vi "Initialise Standard Display.vi"() -> (3 "Standard Display Configuration out":refnum<class "Standard Display Configuration.lvclass">)   [LabVIEW 2016, in "Assert API Components.lvlib" / "Assert Display.lvlib" / "Main Display.lvlib" / "Standard Display Configuration.lvclass"]
uses:
  Standard Display Configuration.lvclass
  Standard Display Configuration.lvclass/Standard Display Configuration.ctl
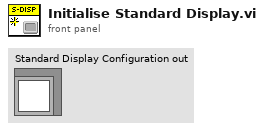
[diagram p1: front panel]
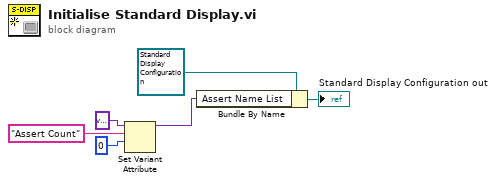
[diagram p0: block diagram]
diagram:
  n1 = Set Variant Attribute(Variant=variant ("Assert Name List"), name="Assert Count", value=0) -> (Variant out=w3:variant)  [unwired: 1 in, 2 out]
  n2 = Bundle By Name(cluster=refnum<class "Standard Display Configuration.lvclass"> refnum ("Standard Display Configuration in"), "Assert Name List"=w3) -> (→"Standard Display Configuration out":refnum<class "Standard Display Configuration.lvclass">)
